vi "Boiler.vi"() -> ()   [LabVIEW 2015]
uses:
  Controls/Boiler Controls.ctl
  Controls/Boiler Simulation Controls.ctl
  Controls/Boiler Status Indicators.ctl
  Controls/status.ctl
  Controls/All data.ctl
  Controls/timer status.ctl
panel:
  out "error out":errorcluster
  in  "error in":errorcluster
  in  "stop":bool
  out "Boiler Status Indicators":T1 {"Time Count" format="%.2g"}
  in  "Boiler Simulation Controls":T2 {"Flame Sensor Value (%)" min=0.0 max=100.0 scale=0.0..100.0}
  in  "Boiler Controls":T3 {"Fuel Valve Position" min=0.0 max=100.0 scale=0.0..100.0 scale format="%.2f"}
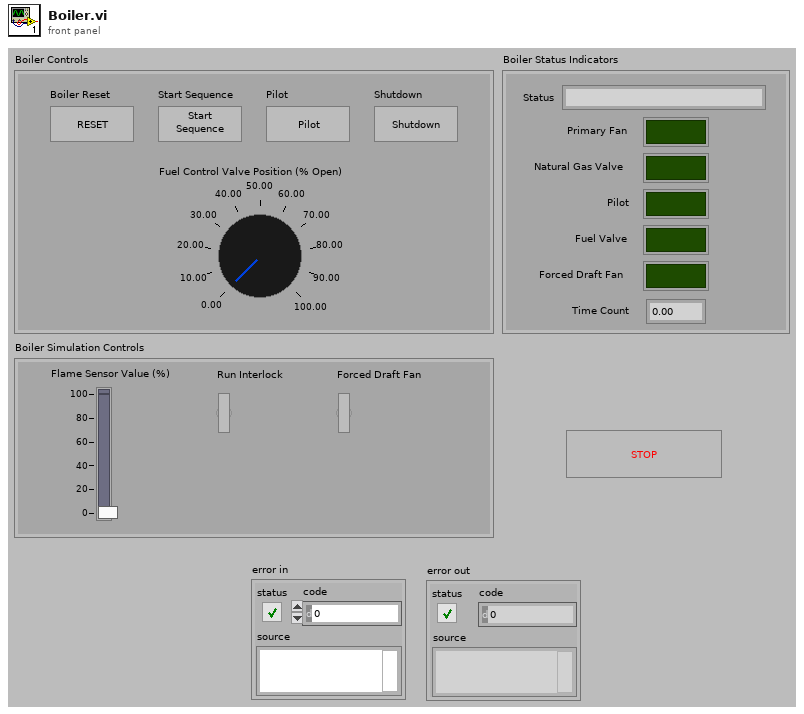
[diagram p1: front panel]
types:
  T1 = typedef "Boiler Status Indicators.ctl" = cluster{"Status":string, "Primary Fan":bool, "Natural Gas Valve":bool, "Pilot":bool, "Fuel Valve":bool, "Forced Draft Fan":bool, "Time Count":dbl}
  T2 = typedef "Boiler Simulation Controls.ctl" = cluster{"Flame Sensor Value (%)":dbl, "Run Interlock":bool, "Forced Draft Fan":bool}
  T3 = typedef "Boiler Controls.ctl" = cluster{"Boiler Reset":bool, "Start Sequence":bool, "Pilot":bool, "Shutdown":bool, "Fuel Valve Position":dbl}
  T4 = typedef "All data.ctl" = cluster{"Log path":path, "Boiler Status Indicators":T1}
  T5 = typedef "status.ctl" = enum16{"Shutdown", "Start&Run-cont", "Start&Run", "Prove Pilot", "Ignition", "Pre Purge-cont", "Pre Purge", "Rerset Lockout", "Start", "Error Under Range", "Exit", "Error", "Idle", "Initialize"}
  T6 = typedef "timer status.ctl" = enum16{"Reset", "Start"}
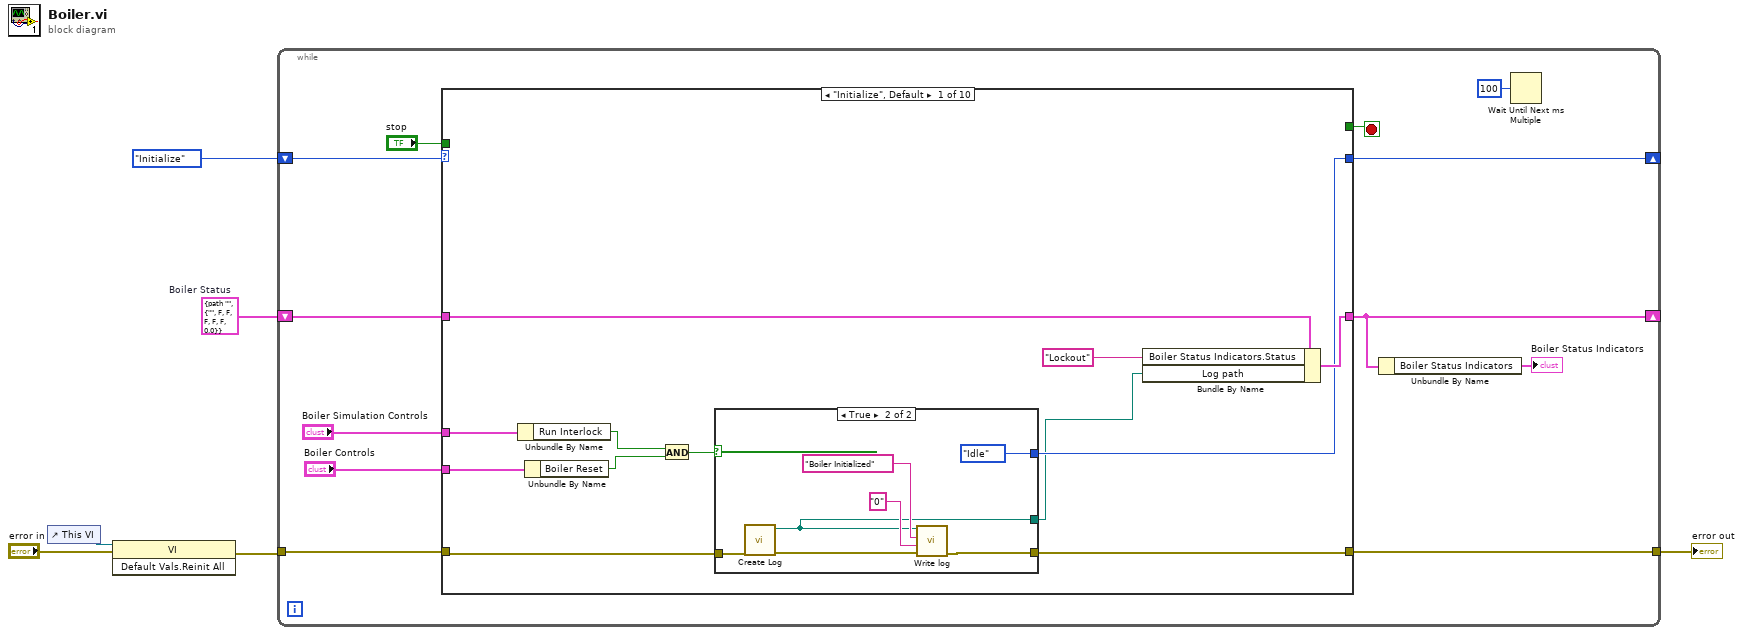
[diagram p0: block diagram]
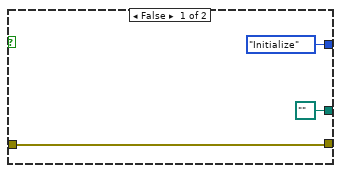
[diagram p2: hidden frame]
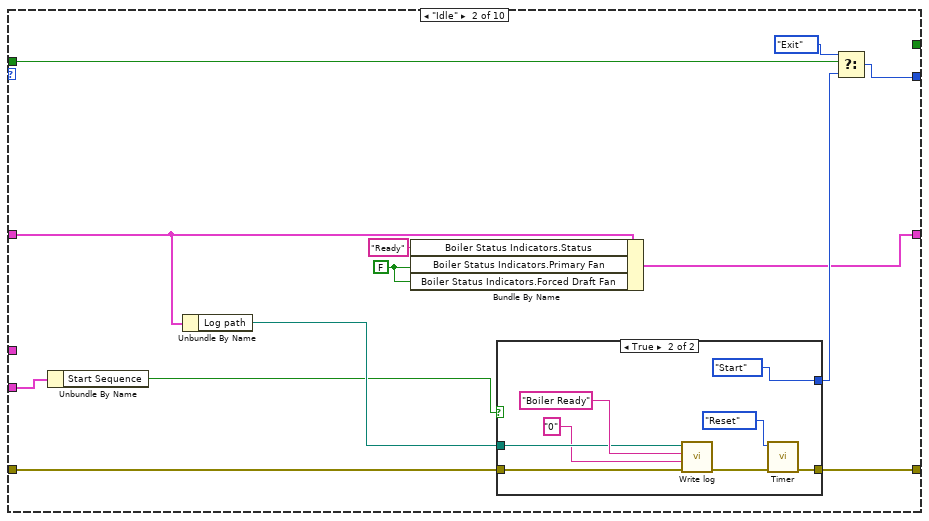
[diagram p3: hidden frame]
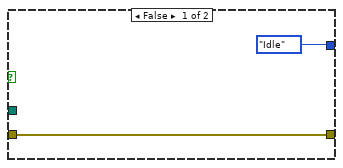
[diagram p4: hidden frame]
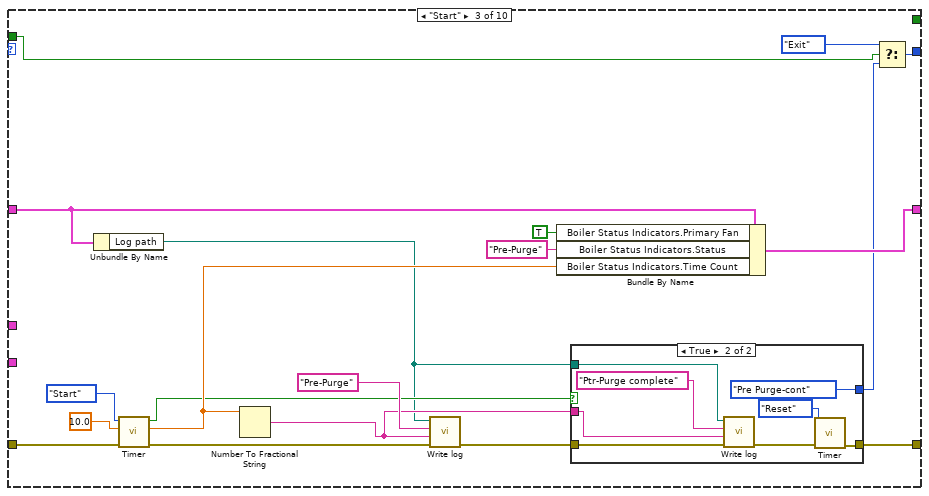
[diagram p5: hidden frame]
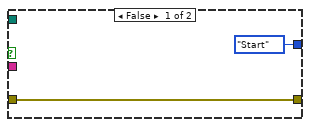
[diagram p6: hidden frame]
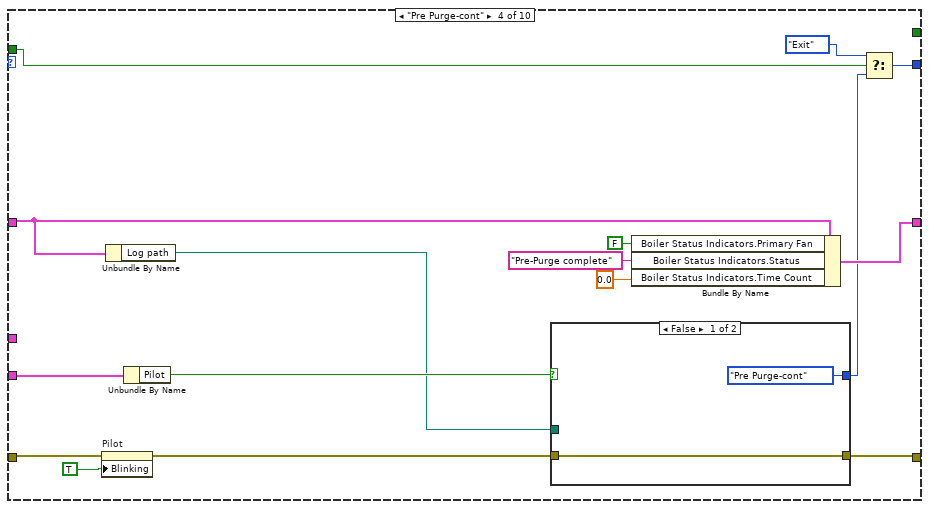
[diagram p7: hidden frame]
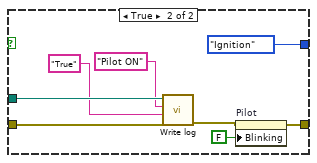
[diagram p8: hidden frame]
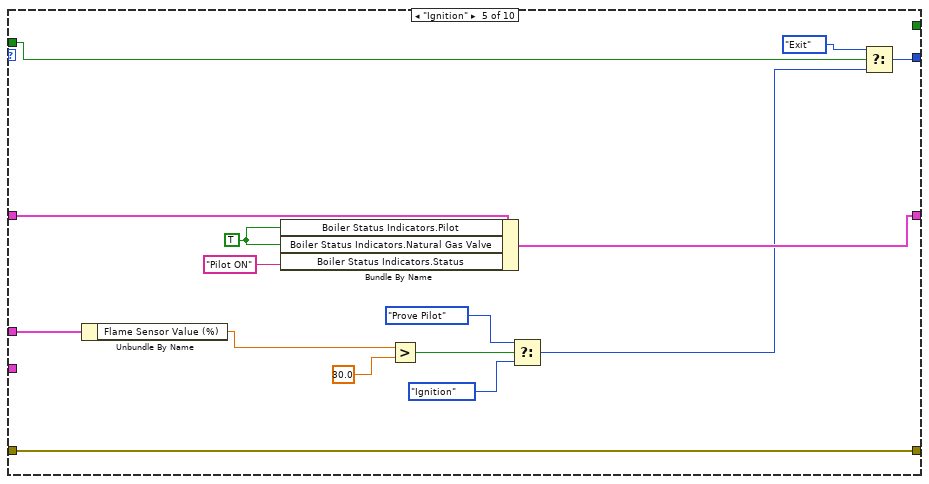
[diagram p9: hidden frame]
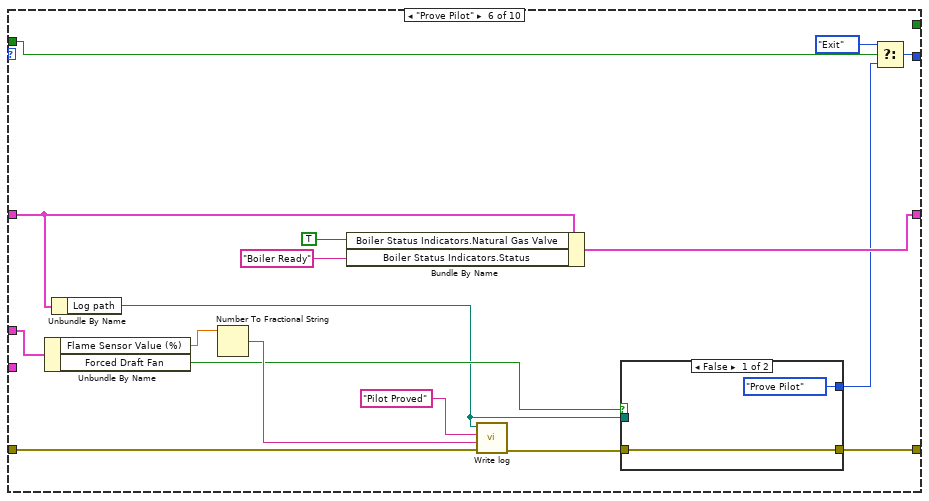
[diagram p10: hidden frame]
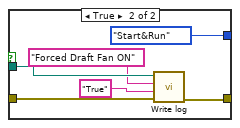
[diagram p11: hidden frame]
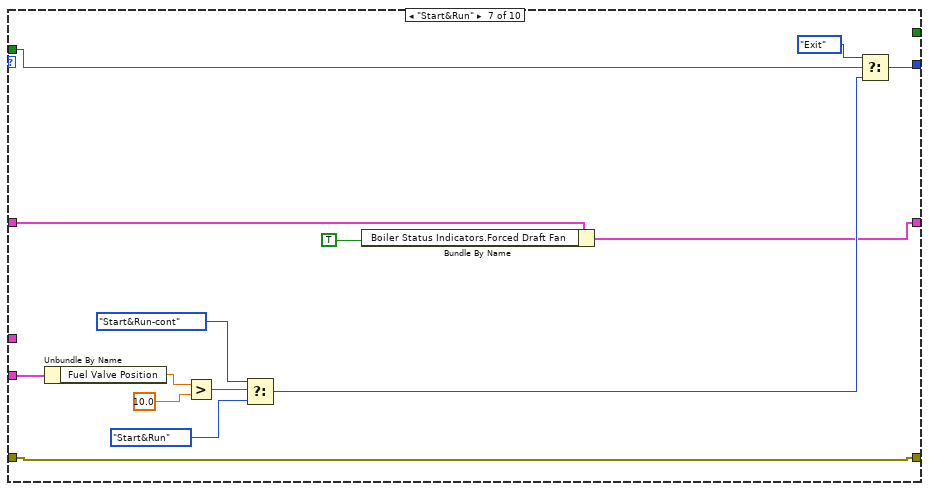
[diagram p12: hidden frame]
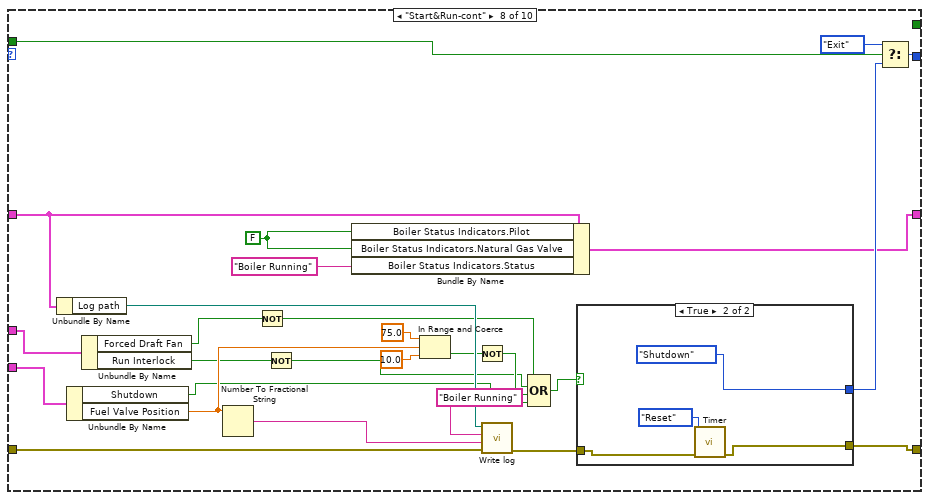
[diagram p13: hidden frame]
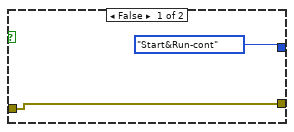
[diagram p14: hidden frame]
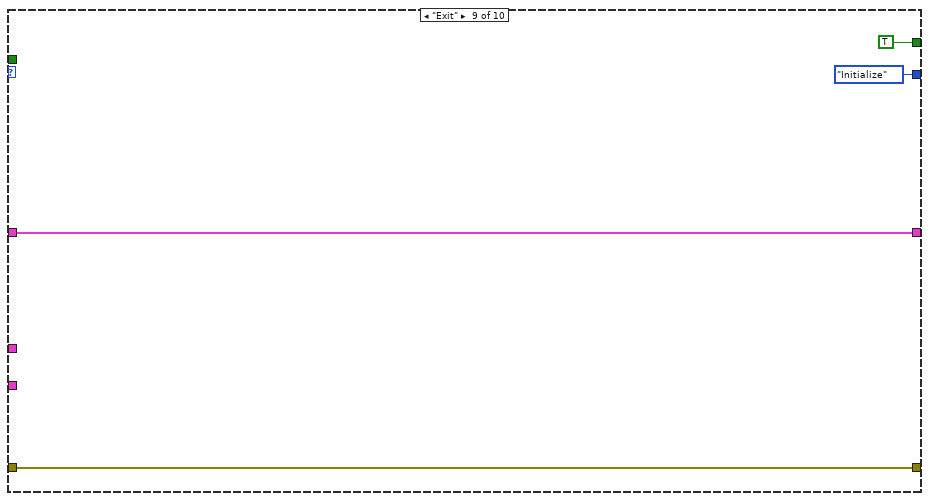
[diagram p15: hidden frame]
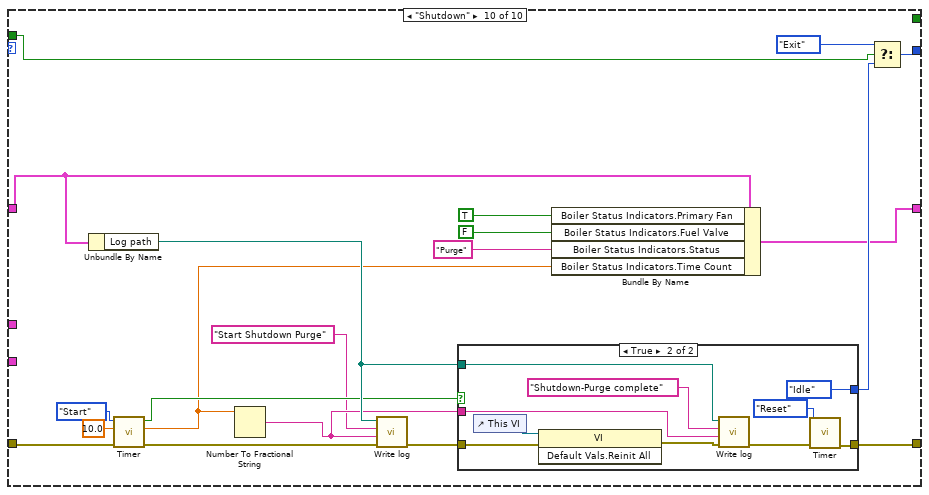
[diagram p16: hidden frame]
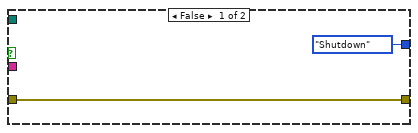
[diagram p17: hidden frame]
diagram:
  w4 = T4 {"Log path"=path "", "Boiler Status Indicators"={"Status"="", "Primary Fan"=FALSE, "Natural Gas Valve"=FALSE, "Pilot"=FALSE, "Fuel Valve"=FALSE, "Forced Draft Fan"=FALSE, "Time Count"=0.0}}  # Boiler Status
  n1 = control-ref of="This VI"() -> (w3:refnum<vi>)
  n2 = invoke class="VI" method="Default Vals.Reinit All"(reference=w3, error in="error in") -> (error out=w1:errorcluster)  [unwired: 1 in, 2 out]
  n3 = while {
    tunnel: w1 -> [w17]
    tunnel: [w16] -> w5
    shift-right: [w13] -> _
    shift-left: w4 -> [w15]
    shift-right: [w14] -> _
    shift-left: status."Initialize" ("status") -> [w18]
    stop <- w8 stop-if-true
    n4 = case shown="\"Initialize\", Default" w18 {
      tunnel: w17 -> [w20 w52 w82 w101 w127 w150 w159 w194 w206 w216]
      tunnel: [w27 w51 w69 w98 w127 w137 w159 w175 w206 w215] -> w16
      tunnel: w15 -> [w30 w45 w77 w105 w133 w142 w162 w193 w207 w213]
      tunnel: [w29 w44 w79 w104 w132 w147 w161 w179 w207 w214] -> w13
      tunnel: [w21 w46 w73 w94 w120 w139 w164 w178 status."Initialize" ("status") w211] -> w14
      tunnel: "Boiler Controls" -> [w25 w53 _ w100 _ _ w172 w192 _ _]
      tunnel: "Boiler Simulation Controls" -> [w26 _ _ _ w130 w145 _ w185 _ _]
      tunnel: "stop" -> [_ w49 w64 w93 w121 w141 w168 w180 _ w210]
      tunnel: [_ _ _ _ _ _ _ _ TRUE _] -> w8
      frame "Initialize", Default {
        n5 = Unbundle By Name(w26) -> ("Run Interlock"=w24:bool)
        n6 = Unbundle By Name(w25) -> ("Boiler Reset"=w23:bool)
        n7 = And(x=w24, y=w23) -> (x .and. y?=w22:bool)
        n8 = case shown="True" w22 {
          tunnel: w20 -> [w33 w36]
          tunnel: [w33 w37] -> w27
          tunnel: [status."Initialize" ("status") status."Idle" ("status")] -> w21
          tunnel: [path "" ("Log path") w34] -> w19
          frame False {
          }
          frame True {
            n9 = call "Create Log.vi"("error in (no error)"=w36) -> ("error out"=w35:errorcluster, "Log path"=w34:path)  [unwired: 9 in]
            n10 = call "Write log.vi"("error in (no error)"=w35, "Event data"="0" ("element"), "Event"="Boiler Initialized" ("element"), "Log path"=w34) -> ("error out"=w37:errorcluster)  [unwired: 7 in]
          }
        }
        n11 = Bundle By Name(cluster=w30, "Boiler Status Indicators.Status"="Lockout" ("Status"), "Log path"=w19) -> (w29:T4)
      }
      frame "Idle" {
        w41 = FALSE ("Boiler Status Indicators.Primary Fan")
        n12 = Unbundle By Name(w53) -> ("Start Sequence"=w42:bool)
        n13 = Unbundle By Name(w45) -> ("Log path"=w50:path)
        n14 = Bundle By Name(cluster=w45, "Boiler Status Indicators.Status"="Ready", "Boiler Status Indicators.Primary Fan"=w41, "Boiler Status Indicators.Forced Draft Fan"=w41) -> (w44:T4)
        n15 = case shown="True" w42 {
          tunnel: w52 -> [w54 w63]
          tunnel: [w54 w57] -> w51
          tunnel: w50 -> [_ w61]
          tunnel: [status."Idle" ("f") status."Start" ("status")] -> w48
          frame False {
          }
          frame True {
            n16 = call "Write log.vi"("error in (no error)"=w63, "Event data"="0", "Event"="Boiler Ready", "Log path"=w61) -> ("error out"=w58:errorcluster)  [unwired: 7 in]
            n17 = call "Timer.vi"("error in"=w58, "timer status"=timer_status."Reset") -> ("error out"=w57:errorcluster)  [unwired: 7 in, 2 out]
          }
        }
        n18 = Select(t=status."Exit", s=w49, f=w48) -> (s? t:f=w46:T5)
      }
      frame "Start" {
        n19 = Unbundle By Name(w77) -> ("Log path"=w66:path)
        n20 = call "Timer.vi"("error in"=w82, "target"=10.0, "timer status"=timer_status."Start") -> ("error out"=w78:errorcluster, "time elapse"=w75:dbl, "elapsed"=w68:bool)  [unwired: 6 in]
        n21 = Number To Fractional String(number=w75) -> (F-format string=w67:string)  [unwired: 3 in]
        n22 = call "Write log.vi"("error in (no error)"=w78, "Event data"=w67, "Event"="Pre-Purge", "Log path"=w66) -> ("error out"=w70:errorcluster)  [unwired: 7 in]
        n23 = Bundle By Name(cluster=w77, "Boiler Status Indicators.Primary Fan"=TRUE, "Boiler Status Indicators.Status"="Pre-Purge", "Boiler Status Indicators.Time Count"=w75) -> (w79:T4)
        n24 = case shown="True" w68 {
          tunnel: w70 -> [w84 w91]
          tunnel: [w84 w87] -> w69
          tunnel: w67 -> [_ w90]
          tunnel: w66 -> [_ w89]
          tunnel: [status."Start" ("status") status."Pre Purge-cont" ("status")] -> w65
          frame False {
          }
          frame True {
            n25 = call "Write log.vi"("error in (no error)"=w91, "Event data"=w90, "Event"="Ptr-Purge complete", "Log path"=w89) -> ("error out"=w86:errorcluster)  [unwired: 7 in]
            n26 = call "Timer.vi"("error in"=w86, "timer status"=timer_status."Reset") -> ("error out"=w87:errorcluster)  [unwired: 7 in, 2 out]
          }
        }
        n27 = Select(t=status."Exit" ("status"), s=w64, f=w65) -> (s? t:f=w73:T5)
      }
      frame "Pre Purge-cont" {
        n28 = property on="Pilot" class="Bool (strict)"(error in=w101, "Blinking"=TRUE) -> (error out=w99:errorcluster)  [unwired: 1 in, 1 out]
        n29 = Unbundle By Name(w105) -> ("Log path"=w96:path)
        n30 = Unbundle By Name(w100) -> ("Pilot"=w97:bool)
        n31 = case shown="False" w97 {
          tunnel: w99 -> [w110 w118]
          tunnel: [w110 w111] -> w98
          tunnel: w96 -> [_ w117]
          tunnel: [status."Pre Purge-cont" ("status") status."Ignition" ("status")] -> w95
          frame False {
          }
          frame True {
            n32 = call "Write log.vi"("error in (no error)"=w118, "Event data"="True", "Event"="Pilot ON", "Log path"=w117) -> ("error out"=w112:errorcluster)  [unwired: 7 in]
            n33 = property on="Pilot" class="Bool (strict)"(error in=w112, "Blinking"=FALSE) -> (error out=w111:errorcluster)  [unwired: 1 in, 1 out]
          }
        }
        n34 = Bundle By Name(cluster=w105, "Boiler Status Indicators.Primary Fan"=FALSE, "Boiler Status Indicators.Status"="Pre-Purge complete", "Boiler Status Indicators.Time Count"=0.0) -> (w104:T4)
        n35 = Select(t=status."Exit" ("status"), s=w93, f=w95) -> (s? t:f=w94:T5)
      }
      frame "Ignition" {
        w119 = TRUE ("Boiler Status Indicators.Natural Gas Valve")
        n36 = Unbundle By Name(w130) -> ("Flame Sensor Value (%)"=w129:dbl)
        n37 = Bundle By Name(cluster=w133, "Boiler Status Indicators.Pilot"=w119, "Boiler Status Indicators.Natural Gas Valve"=w119, "Boiler Status Indicators.Status"="Pilot ON") -> (w132:T4)
        n38 = Greater?(x=w129, y=30.0) -> (0:w125:bool)
        n39 = Select(t=status."Prove Pilot" ("status"), s=w125, f=status."Ignition" ("status")) -> (s? t:f=w122:T5)
        n40 = Select(t=status."Exit" ("status"), s=w121, f=w122) -> (s? t:f=w120:T5)
      }
      frame "Prove Pilot" {
        n41 = Unbundle By Name(w145) -> ("Flame Sensor Value (%)"=w144:dbl, "Forced Draft Fan"=w136:bool)
        n42 = Unbundle By Name(w142) -> ("Log path"=w135:path)
        n43 = Number To Fractional String(number=w144) -> (F-format string=w143:string)  [unwired: 3 in]
        n44 = Bundle By Name(cluster=w142, "Boiler Status Indicators.Natural Gas Valve"=TRUE, "Boiler Status Indicators.Status"="Boiler Ready") -> (w147:T4)
        n45 = call "Write log.vi"("error in (no error)"=w150, "Event data"=w143, "Event"="Pilot Proved", "Log path"=w135) -> ("error out"=w138:errorcluster)  [unwired: 7 in]
        n46 = case shown="False" w136 {
          tunnel: [w151 w157] -> w137
          tunnel: w138 -> [w151 w158]
          tunnel: w135 -> [_ w156]
          tunnel: [status."Prove Pilot" ("status") status."Start&Run" ("status")] -> w134
          frame False {
          }
          frame True {
            n47 = call "Write log.vi"("error in (no error)"=w158, "Event data"="True", "Event"="Forced Draft Fan ON", "Log path"=w156) -> ("error out"=w157:errorcluster)  [unwired: 7 in]
          }
        }
        n48 = Select(t=status."Exit", s=w141, f=w134) -> (s? t:f=w139:T5)
      }
      frame "Start&Run" {
        n49 = Unbundle By Name(w172) -> ("Fuel Valve Position"=w171:dbl)
        n50 = Greater?(x=w171, y=10.0) -> (0:w169:bool)
        n51 = Select(t=status."Start&Run-cont" ("status"), s=w169, f=status."Start&Run" ("status")) -> (s? t:f=w165:T5)
        n52 = Bundle By Name(cluster=w162, "Boiler Status Indicators.Forced Draft Fan"=TRUE) -> (w161:T4)
        n53 = Select(t=status."Exit", s=w168, f=w165) -> (s? t:f=w164:T5)
      }
      frame "Start&Run-cont" {
        w191 = FALSE ("Boiler Status Indicators.Natural Gas Valve")
        n54 = Unbundle By Name(w193) -> ("Log path"=w199:path)
        n55 = Unbundle By Name(w192) -> ("Shutdown"=w182:bool, "Fuel Valve Position"=w188:dbl)
        n56 = Unbundle By Name(w185) -> ("Forced Draft Fan"=w184:bool, "Run Interlock"=w183:bool)
        n57 = Number To Fractional String(number=w188) -> (F-format string=w197:string)  [unwired: 3 in]
        n58 = Not(x=w184) -> (.not. x?=w176:bool)
        n59 = Not(x=w183) -> (.not. x?=w177:bool)
        n60 = Bundle By Name(cluster=w193, "Boiler Status Indicators.Pilot"=w191, "Boiler Status Indicators.Natural Gas Valve"=w191, "Boiler Status Indicators.Status"="Boiler Running") -> (w179:T4)
        n61 = In Range and Coerce(upper limit=75.0, x=w188, lower limit=10.0) -> (In Range?=w186:bool)  [unwired: 1 out]
        n62 = Not(x=w186) -> (.not. x?=w187:bool)
        n63 = call "Write log.vi"("error in (no error)"=w194, "Event data"=w197, "Event"="Boiler Running", "Log path"=w199) -> ("error out"=w174:errorcluster)  [unwired: 7 in]
        n64 = Compound Arithmetic op=OR(w176, w177, w187, w182) -> (w173:bool)
        n65 = case shown="True" w173 {
          tunnel: [status."Start&Run-cont" ("t") status."Shutdown" ("t")] -> w181
          tunnel: [w200 w203] -> w175
          tunnel: w174 -> [w200 w204]
          frame False {
          }
          frame True {
            n66 = call "Timer.vi"("error in"=w204, "timer status"=timer_status."Reset") -> ("error out"=w203:errorcluster)  [unwired: 7 in, 2 out]
          }
        }
        n67 = Select(t=status."Exit", s=w180, f=w181) -> (s? t:f=w178:T5)
      }
      frame "Exit" {
      }
      frame "Shutdown" {
        n68 = Unbundle By Name(w213) -> ("Log path"=w228:path)
        n69 = call "Timer.vi"("error in"=w216, "target"=10.0, "timer status"=timer_status."Start") -> ("error out"=w219:errorcluster, "time elapse"=w221:dbl, "elapsed"=w226:bool)  [unwired: 6 in]
        n70 = Number To Fractional String(number=w221) -> (F-format string=w227:string)  [unwired: 3 in]
        n71 = call "Write log.vi"("error in (no error)"=w219, "Event data"=w227, "Event"="Start Shutdown Purge", "Log path"=w228) -> ("error out"=w225:errorcluster)  [unwired: 7 in]
        n72 = case shown="True" w226 {
          tunnel: w225 -> [w231 w233]
          tunnel: [w231 w237] -> w215
          tunnel: w227 -> [_ w240]
          tunnel: w228 -> [_ w239]
          tunnel: [status."Shutdown" ("status") status."Idle" ("status")] -> w229
          frame False {
          }
          frame True {
            n73 = control-ref of="This VI"() -> (w234:refnum<vi>)
            n74 = invoke class="VI" method="Default Vals.Reinit All"(reference=w234, error in=w233) -> (error out=w232:errorcluster)  [unwired: 1 in, 2 out]
            n75 = call "Write log.vi"("error in (no error)"=w232, "Event data"=w240, "Event"="Shutdown-Purge complete", "Log path"=w239) -> ("error out"=w236:errorcluster)  [unwired: 7 in]
            n76 = call "Timer.vi"("error in"=w236, "timer status"=timer_status."Reset") -> ("error out"=w237:errorcluster)  [unwired: 7 in, 2 out]
          }
        }
        n77 = Bundle By Name(cluster=w213, "Boiler Status Indicators.Primary Fan"=TRUE, "Boiler Status Indicators.Fuel Valve"=FALSE ("Boiler Status Indicators.Primary Fan"), "Boiler Status Indicators.Status"="Purge", "Boiler Status Indicators.Time Count"=w221) -> (w214:T4)
        n78 = Select(t=status."Exit" ("status"), s=w210, f=w229) -> (s? t:f=w211:T5)
      }
    }
    n79 = Unbundle By Name(w13) -> ("Boiler Status Indicators"=→"Boiler Status Indicators":T1)
    n80 = Wait Until Next ms Multiple(millisecond multiple=u32 100) -> ()  [unwired: 1 out]
  }
  "error out" <- w5
